vi "get set udp value from dev var alias array.vi"(6 "slow timeout ms (3000)":i32=3000, 8 "error in (no error)":errorcluster, 9 "Set position":dbl, 10 "get or set":enum16{"get", "set"}(ring), 11 "device and variable":string[](array[string])) -> (0 "error out":errorcluster, 2 "No errors =T":bool, 3 "Numeric":dbl)   [LabVIEW 2020]
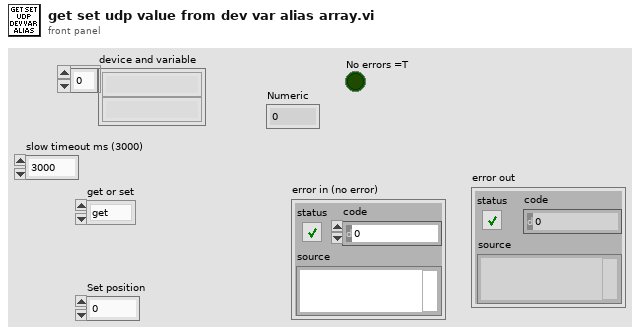
[diagram p1: front panel]
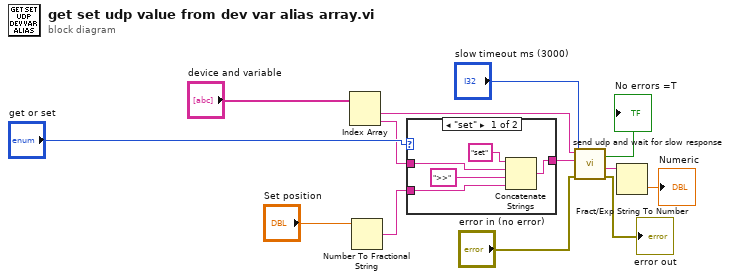
[diagram p0: block diagram]
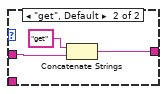
[diagram p2: hidden frame]
diagram:
  n1 = Index Array(array="device and variable") -> (element #1=w10:string, element #2=w9:string)  [unwired: 2 in]
  n2 = Number To Fractional String(number="Set position") -> (F-format string=w12:string)  [unwired: 3 in]
  n3 = case shown="\"set\"" "get or set" {
    tunnel: [w16 w20] -> w8
    tunnel: w9 -> [w15 w19]
    tunnel: w12 -> [w14 _]
    frame "set" {
      n4 = Concatenate Strings("set" ("command in"), w15, ">>" ("string"), w14) -> (w16:string)
    }
    frame "get", Default {
      n5 = Concatenate Strings("get" ("command in"), w19) -> (w20:string)
    }
  }
  n6 = call "send udp and wait for slow response.vi"("error in"="error in (no error)", "slow timeout ms (3000)"="slow timeout ms (3000)", "command in"=w8, "Device"=w10) -> ("error out"=→"error out":errorcluster, "value for real"=w7:string, "No errors"=→"No errors =T":bool)  [unwired: 3 in, 2 out]
  n7 = Fract/Exp String To Number(string=w7) -> (number=→"Numeric":dbl)  [unwired: 3 in, 1 out]
